vi "04 Occurences and more.vi"() -> ()   [LabVIEW 2019]
panel:
  out "Current Loop 1":i32
  out "Total Fired":u8
  out "Total Occurrences Fired":u8
  out "Current Loop 1 Iteration":i32
  in  "Stop":bool
  # "Hit the Run arrow and see the Gauge change to the value of the Slide\n\nHit Continuous Run and watch the Gauge change as you vary the Slide"
  # "Hit Cmd E to see the diagram (code)"
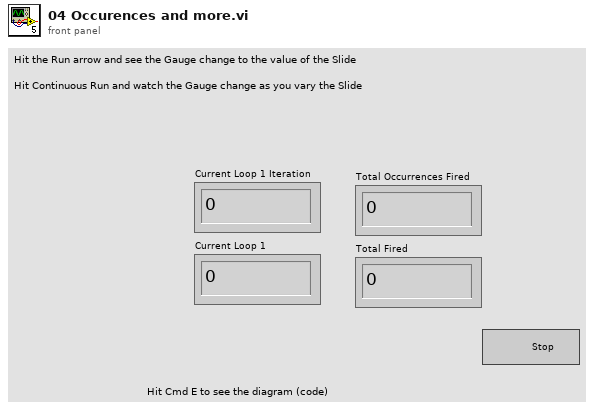
[diagram p1: front panel]
types:
  T1 = typedef "Semaphore RefNum" = refnum<k1>
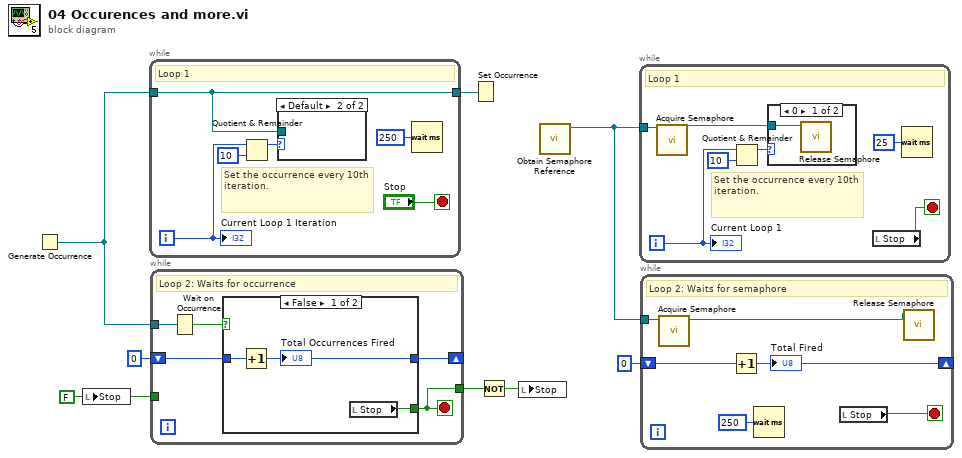
[diagram p0: block diagram]
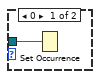
[diagram p4: hidden frame]
diagram:
  w3 = FALSE ("Loop Stop")
  n1 = Generate Occurrence() -> (w8:refnum<k4>)
  n2 = local write "Stop"(w3) -> ()
  n3 = while {
    tunnel: w8 -> [w12]
    tunnel: [w12] -> w7
    i -> [w9]
    stop <- "Stop" stop-if-true
    # "Set the occurrence every 10th iteration."
    # "Loop 1"
    n4 = Quotient & Remainder(x=w9, y=10) -> (x-y*floor(x/y)=w13:i32)  [unwired: 1 out]
    n5 = case shown="Default" w13 {
      tunnel: w12 -> [w15 _]
      frame 0 {
        n6 = Set Occurrence(w15) -> ()
      }
      frame Default {
      }
    }
    n7 = Wait (ms)(milliseconds to wait=u32 250) -> ()  [unwired: 1 out]
    "Current Loop 1 Iteration" <- w9
  }
  n8 = while {
    tunnel: w8 -> [w20]
    shift-right: [w17] -> _
    shift-left: u8 0 -> [w18]
    tunnel: [w16] -> w5
    tunnel: w3 -> [_]
    stop <- w16 stop-if-true
    # "Loop 2: Waits for occurrence"
    n9 = Wait on Occurrence(2:w20) -> (0:w19:bool)  [unwired: 2 in]
    n10 = case shown="False" w19 {
      tunnel: [w21 _] -> w16
      tunnel: w18 -> [w23 w24]
      tunnel: [w22 w24] -> w17
      frame False {
        n11 = Increment(x=w23) -> (x+1=w22:u8)
        "Total Occurrences Fired" <- w22
        n12 = local read "Stop"() -> (w21:bool)
      }
      frame True {
      }
    }
  }
  n13 = Set Occurrence(w7) -> ()
  n14 = Not(x=w5) -> (.not. x?=w4:bool)
  n15 = local write "Stop"(w4) -> ()
  n16 = call <vilib>:"Obtain Semaphore Reference.vi"() -> ("semaphore"=w1:T1)  [unwired: 5 in, 2 out]
  n17 = while {
    tunnel: w1 -> [w27]
    i -> [w28]
    stop <- w25 stop-if-true
    # "Set the occurrence every 10th iteration."
    # "Loop 1"
    n18 = call <vilib>:"Acquire Semaphore.vi"("semaphore"=w27) -> ("semaphore out"=w26:T1)  [unwired: 4 in, 2 out]
    n19 = Quotient & Remainder(x=w28, y=10) -> (x-y*floor(x/y)=w30:i32)  [unwired: 1 out]
    n20 = case shown="0" w30 {
      tunnel: w26 -> [w32 _]
      frame 0 {
        n21 = call <vilib>:"Release Semaphore.vi"("semaphore"=w32) -> ()  [unwired: 5 in, 2 out]
      }
      frame Default {
      }
    }
    n22 = local read "Stop"() -> (w25:bool)
    n23 = Wait (ms)(milliseconds to wait=u32 25) -> ()  [unwired: 1 out]
    "Current Loop 1" <- w28
  }
  n24 = while {
    shift-right: [w37] -> _
    shift-left: u8 0 -> [w38]
    tunnel: w1 -> [w35]
    stop <- w36 stop-if-true
    # "Loop 2: Waits for semaphore"
    n25 = call <vilib>:"Acquire Semaphore.vi"("semaphore"=w35) -> ("semaphore out"=w33:T1)  [unwired: 4 in, 2 out]
    n26 = Increment(x=w38) -> (x+1=w37:u8)
    "Total Fired" <- w37
    n27 = Wait (ms)(milliseconds to wait=u32 250) -> ()  [unwired: 1 out]
    n28 = local read "Stop"() -> (w36:bool)
    n29 = call <vilib>:"Release Semaphore.vi"("semaphore"=w33) -> ()  [unwired: 5 in, 2 out]
  }
